vi "Syncing.vi"(7 "Stop Reference":refnum<vi>, 9 "Counters":tag[](array[tag])=["Dev1/ctr0", "Dev1/ctr1"], 10 "Sample Lines":tag[](array[tag])=["/Dev1/PFI0", "/Dev1/PFI1", "/Dev1/PFI2", "/Dev1/PFI3", "/Dev1/PFI4", "/Dev1/PFI5", "/Dev1/PFI6", "/Dev1/PFI7"], 11 "Counters":i32=2) -> (3 "Timestamps":u64[][](array[numeric]))   [LabVIEW 2010]
uses:
  <vilib>/DAQmx/write.llb/DAQmx Write (Digital Bool 1Line 1Point).vi
  <vilib>/DAQmx/read.llb/DAQmx Read (Counter U32 1Chan 1Samp).vi
  <vilib>/DAQmx/create/channels.llb/DAQmx Create Channel (DO-Digital Output).vi
  <vilib>/DAQmx/create/channels.llb/DAQmx Create Channel (CI-Count Edges).vi
  <vilib>/DAQmx/configure/timing.llb/DAQmx Timing (Sample Clock).vi
  <vilib>/daqmx/miscellaneous.llb/DAQmx Fill In Error Info.vi
  Program Files/National Instruments/LabVIEW 2010/resource/objmgr/daqmx.rc
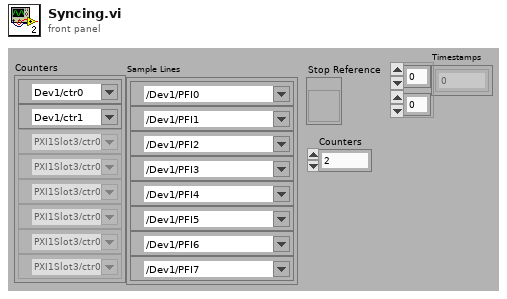
[diagram p1: front panel]
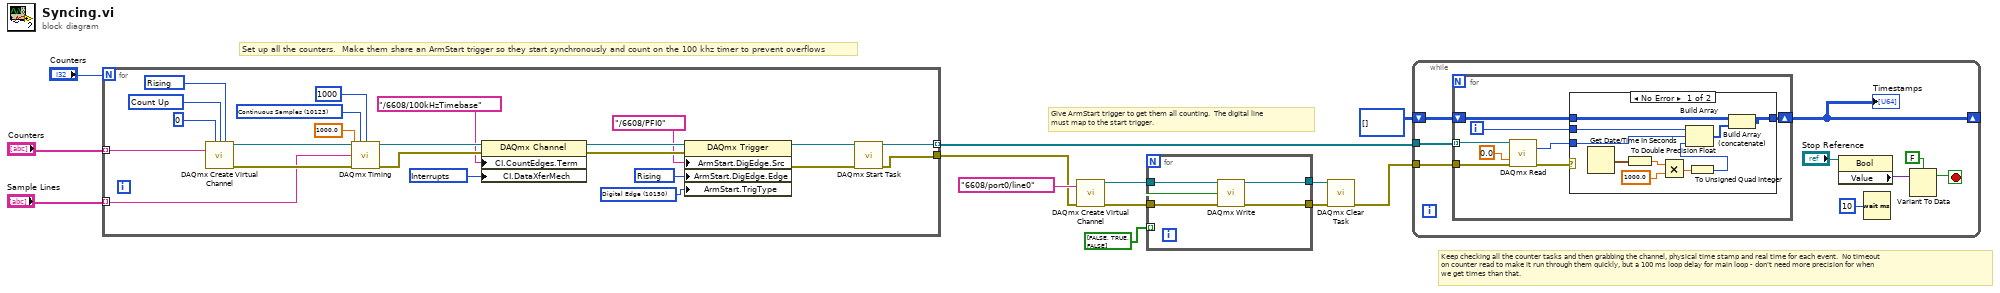
[diagram p0: block diagram]
diagram:
  # "Keep checking all the counter tasks and then grabbing the channel, physical time stamp and real time for each event.  No timeout\non counter read to make it run through them quickly, but a 100 ms loop delay for main loop - don't need more precision for when\nwe get times than that."
  # "Give ArmStart trigger to get them all counting.  The digital line\nmust map to the start trigger."
  # "Set up all the counters.  Make them share an ArmStart trigger so they start synchronously and count on the 100 khz timer to prevent overflows"
  n1 = for {
    N: "Counters" -> [_]
    tunnel: "Counters" -> [w33] mode=indexing
    tunnel: [w27] -> w12 mode=indexing
    tunnel: [w26] -> w7
    tunnel: "Sample Lines" -> [w17] mode=indexing
    w15 = 10204 items=["DMA"=10054, "Interrupts"=10204, "Programmed I/O"=10264, "USB Bulk"=12590] ("CI.DataXferMech")
    w18 = 10150 items=["Digital Edge"=10150, "None"=10230] ("ArmStart.TrigType")
    w19 = 10280 items=["Rising"=10280, "Falling"=10171] ("ArmStart.DigEdge.Edge")
    w30 = 10123 items=["Finite Samples"=10178, "Continuous Samples"=10123, "Hardware Timed Single Point"=12522] ("sample mode")
    w34 = 10280 items=["Rising"=10280, "Falling"=10171] ("edge")
    w35 = 10128 items=["Count Up"=10128, "Count Down"=10124, "Externally Controlled"=10326] ("count direction")
    n2 = call-poly <vilib>:"DAQmx Create Virtual Channel.vi"("initial count"=0, "count direction"=w35, "edge"=w34, "counter"=w33) -> ("task out"=w32:refnum<k21>, "error out"=w31:errorcluster)  [unwired: 10 in]
    n3 = call-poly <vilib>:"DAQmx Timing.vi"("task/channels in"=w32, "sample mode"=w30, "samples per channel"=1000, "rate"=1000.0, "source"=w17, "error in"=w31) -> ("task out"=w22:refnum<k21>, "error out"=w23:errorcluster)  [unwired: 8 in]
    n4 = property class="DAQmx Channel"(reference=w22, error in=w23, "CI.CountEdges.Term"=tag "/6608/100kHzTimebase", "CI.DataXferMech"=w15) -> (reference out=w21:refnum<k21>, error out=w20:errorcluster)
    n5 = property class="DAQmx Trigger"(reference=w21, error in=w20, "ArmStart.DigEdge.Src"=tag "/6608/PFI0" ("Start Trigger"), "ArmStart.DigEdge.Edge"=w19, "ArmStart.TrigType"=w18) -> (reference out=w25:refnum<k21>, error out=w24:errorcluster)
    n6 = call <vilib>:"DAQmx Start Task.vi"("task/channels in"=w25, "error in"=w24) -> ("task out"=w27:refnum<k21>, "error out"=w26:errorcluster)  [unwired: 12 in]
  }
  n7 = call-poly <vilib>:"DAQmx Create Virtual Channel.vi"("lines"=tag "6608/port0/line0", "error in"=w7) -> ("task out"=w10:refnum<k21>, "error out"=w9:errorcluster)  [unwired: 12 in]
  n8 = for {
    tunnel: w10 -> [w41]
    tunnel: w9 -> [w40]
    tunnel: [w39] -> w5
    tunnel: [w38] -> w6
    tunnel: bool[] [FALSE, TRUE, FALSE] -> [w37] mode=indexing
    n9 = call-poly <vilib>:"DAQmx Write.vi"("task/channels in"=w41, "data"=w37, "error in"=w40) -> ("task out"=w39:refnum<k21>, "error out"=w38:errorcluster)  [unwired: 10 in, 1 out]
  }
  n10 = call <vilib>:"DAQmx Clear Task.vi"("task in"=w5, "error in"=w6) -> ("error out"=w3:errorcluster)  [unwired: 13 in]
  n11 = while {
    tunnel: w12 -> [w50]
    tunnel: w3 -> [w49]
    shift-right: [w48] -> _
    shift-left: u64[][] [] -> [w47]
    stop <- w43 stop-if-true
    n12 = for {
      tunnel: w50 -> [w58] mode=indexing
      tunnel: w49 -> [w57]
      shift-right: [w53] -> w48
      shift-left: w47 -> [w51]
      i -> [w55]
      n13 = call-poly <vilib>:"DAQmx Read.vi"("task/channels in"=w58, "timeout"=0.0, "error in"=w57) -> ("data"=w54:u32, "error out"=w52:errorcluster)  [unwired: 10 in, 1 out]
      n14 = case shown="No Error" w52 {
        tunnel: w55 -> [w68 _]
        tunnel: w54 -> [w67 _]
        tunnel: w51 -> [w66 w69]
        tunnel: [w65 w69] -> w53
        frame No Error {
          n15 = Get Date/Time In Seconds() -> (seconds since 1Jan1904=w63:timestamp)
          n16 = To Double Precision Float(number=w63) -> (double precision float=w62:dbl)
          n17 = Multiply(x=w62, y=1000.0) -> (x*y=w60:dbl)
          n18 = To Unsigned Quad Integer(1:w60) -> (0:w59:u64)
          n19 = Build Array(w68, w67, w59) -> (w64:u64[])
          n20 = Build Array (concatenate)(w66, w64) -> (w65:u64[][])
        }
        frame Error {
        }
      }
    }
    "Timestamps" <- w48
    n21 = property class="Bool"(reference="Stop Reference") -> ("Value"=w45:variant)  [unwired: 1 in, 2 out]
    n22 = Wait (ms)(milliseconds to wait=u32 10) -> ()  [unwired: 1 out]
    n23 = Variant To Data(Variant=w45, type=FALSE) -> (data=w43:bool)  [unwired: 1 in, 1 out]
  }
